vi "GPS_Air530Browser.vi"() -> ()   [LabVIEW 2024]
uses:
  <vilib>/sklein/WebView2/Webview2 Control/WebView2 Control.xctl
  Driver/CTIPicoVISA.lvlib
panel:
  out "WebView2 Control":string(xcontrol)
  out "Url":string
  out "Time Stamp":timestamp format="%<%.3X>T"
  out "Longitude":dbl format="%#_12f"
  out "Latitude":dbl format="%#_12f"
  out "$GNGGA":string
  out "error out":errorcluster
  out "NMEA Data":string="$GNGGA,100842.000,5113.89397,N,00120.47732,W,1,18,0.6,78.5,M,47.2,M,,*67\r\n$GNGLL,5113.89397,N,00120.47732,W,100842.000,A,A*56\r\n$GNGSA,A,3,01,02,03,08,10,14,17,22,27,32,,,1.0,0.6,0.8,1*30\r\n$GNGSA,A,3,12,19,20,21,22,34,35,44,,,,,1.0,0.6,0.8,4*30\r\n$GPGSV,3,1,10,01,73,289,48,02,73,0843,03,44221,35,19\r\n$PGSV,3,211,027,283,49,1722,26,302,44GPGSV,3,3,10,27,05,148,26,32,33,062,38,0*63\r\n$BDGSV,2,1,08,12,51,298,43,19,50,067,40,20,10,037,28,21,09,199,31,0*70\r\n$BDGSV,2,2,08,22,52,166,44,34,23,299,44,35,50,128,38,44,78,278,43,0*78\r\n$GNRMC,100842.000,A,5113.89397,N,00120.47732,W,0.00,0.00,130725,,,A,V*19\r\n$GNVTG,0.00,T,,M,0.00,N,0.00,K,A*23\r\n$GNZDA,100842.000,13,07,2025,00,00*47\r\n$GPTXT,01,01,01,ANTENNA OK*35\r\n$GNGGA,100843.000,5113.89397,N,00120.47732,W,1,18,0.6,78.5,M,47.2,M,,*66\r\n$GNGLL,5113.89397,N,00120.47732,W,100843.000,A,A*57\r\n$GNGSA,A,3,01,02,03,08,10,14,17,22,27,32,,,1.0,0.6,0.8,1*30\r\n$GNGSA,A,3,12,19,20,21,22,34,35,44,,,,,1.0,0.6,0.8,4*30\r\n$GPGSV,3,1,10,01,73,289,48,02,73,087,43,03,44,221,34,08,35,162,41,0*69\r\n$GPGSV,3,2,10,10,11,052,27,14,27,283,49,17,27,309,42,22,26,302,44,0*68\r\n$GPGSV,3,3,10,27,05,148,26,32,33,062,38,0*63\r\n$BDGSV,2,1,08,12,51,298,43,19,50,067,41,20,10,037,28,21,09,199,31,0*71\r\n$BDGSV,2,2,08,22,52,166,44,34,23,299,44,35,50,128,38,44,78,278,43,0*78\r\n$GNRMC,100843.000,A,5113.89397,N,00120.47732,W,0.00,0.00,130725,,,A,V*18\r\n$GNVTG,0.00,T,,M,0.00,N,0.00,K,A*23\r\n$GNZDA,100843.000,13,07,2025,00,00*46\r\n$GPTXT,01,01,01,ANTENNA OK*35\r\n$GNGGA,100844.000,5113.89397,N,00120.47732,W,1,18,0.6,78.5,M,47.2,M,,*61\r\n$GNGLL,5113.89397,N,00120.47732,W,100844.000,A,A*50\r\n$GNGSA,A,3,01,02,03,08,10,14,17,22,27,32,,,1.0,0.6,0.8,1*30\r\n$GNGSA,A,3,12,19,20,21,22,34,35,44,,,,,1.0,0.6,0.8,4*30\r\n$GPGSV,3,1,10,01,73,289,48,02,73,087,43,03,44,221,34,08,35,162,41,0*69\r\n$GPGSV,3,2,10,10,11,052,27,14,27,283,49,17,27,309,43,22,26,302,44,0*69\r\n$GPGSV,3,3,10,27,05,148,26,32,33,062,38,0*63\r\n$BDGSV,2,1,08,12,51,298,43,19,50,067,41,20,10,037,28,21,09,199,30,0*70\r\n$BDGSV,2,2,08,22,52,166,44,34,23,299,44,35,50,128,38,44,78,278,42,0*79\r\n$GNRMC,100844.000,A,5113.89397,N,00120.47732,W,0.00,0.00,130725,,,A,V*1F\r\n$GNVTG,0.00,T,,M,0.00,N,0.00,K,A*23\r\n$GNZDA,100844.000,13,07,2025,00,00*41\r\n$GPTXT,01,01,01,ANTENNA OK*35\r\n$GNGGA,100845.000,5113.89397,N,00120.47732,W,1,18,0.6,78.5,M,47.2,M,,*60\r\n$GNGLL,5113.89397,N,00120.47732,W,100845.000,A,A*51\r\n$GNGSA,A,3,01,02,03,08,10,14,17,22,27,32,,,1.0,0.6,0.8,1*30\r\n$GNGSA,A,3,12,19,20,21,22,34,35,44,,,,,1.0,0.6,0.8,4*30\r\n$GPGSV,3,1,10,01,73,289,48,02,73,087,43,03,44,221,34,08,35,162,41,0*69\r\n$GPGSV,3,2,10,10,11,052,24,14,27,283,49,17,27,309,43,22,26,302,44,0*6A\r\n$GPGSV,3,3,10,27,05,148,26,32,33,062,38,0*63\r\n$BDGSV,2,1,08,12,51,298,43,19,50,067,41,20,10,037,28,21,09,199,30,0*70\r\n$BDGSV,2,2,08,22,52,166,44,34,23,299,44,35,50,128,38,44,78,278,42,0*79\r\n$GNRMC,100845.000,A,5113.89397,N,00120.47732,W,0.00,0.00,130725,,,A,V*1E\r\n$GNVTG,0.00,T,,M,0.00,N,0.00,K,A*23\r\n$GNZDA,100845.000,13,07,202500*4PTXT01,01,01A OK*35\r$GNGGA,100846.000,5113.89397,N,00120.47732,W,1,18,0.6,78.5,M,47.2,M,,*63GLL,5113.89320.47732,W,10084A,A*52\r\nA,3,01,02,03,17,22,27,32,,,1.8,1*30\r\n$GNGSA,12,19,204,35,44,,,,,1.0,0.8,4*30V,3,1,10,01,73,28,02,73,087,43,0221,34,02,41,0*69\r\n$GPGS,10,10,124,14,27,17,309,302,44,0*6A\r\n$GP3,3,10,232,33,062,3863\r\nGSV,2,51,2989,50067,41,27,28,21,09,130,00\r\n$BDGS08,22,52,299,43,35,538,44,78,278\r\n$GNRMC,100,A,5113.89397,N,.47732,W0725,,A,V*1DG,0.00,T,,M,.00,K,A*23\r\n$GNZ.000,13,07,20*43\n$GPTXT,01,01,01,ANTENNA OK*35\r\n$GNGGA,100847.000,5113.89397,N,00120.47732,W,1,18,0.,78.2\r\n$113.10087.00,A,A3,0102,03,087,320.6,2,191,22.0,06,0.1,1001,72,73,34,3,2,17,2,05,12,598,4,27,09,1GSV,,299,35,3,0*\n$GN511397,N.00,*1C\rGNVTG,0.\r\n$GZDA,008400,001,0,ANT\r\n$GNGGA,100848.000,5113.89398,N,00120.47731W,1,,0.678.5GNGL20.4731,,100$GNG,14,7,2227,3GSA,3,1244,,0,0.V,3,,10,73,0,1621,0*3,2,50,1,27,0*60\n$GPSV,332,3,06238,098,419,57,2109,19,28,08,3,293,3578,448.0A,51,W,000,0NVTG0.0023\r\n00*4$GPT*35\r$GNGGA,1"
  in  "Len (LineTerm)":u8=4
  in  "UART Connector":enum16{"UART0", "UART1"}(ring)=enum."UART1"
  out "Identity":T1
  in  "Term Char (None)":string
  in  "Baud":u32=9600
  in  "VISA resource name in":refnum<visa-resource-name>
  in  "stop":bool
  # "https://wiki.seeedstudio.com/Grove-GPS-Air530/"
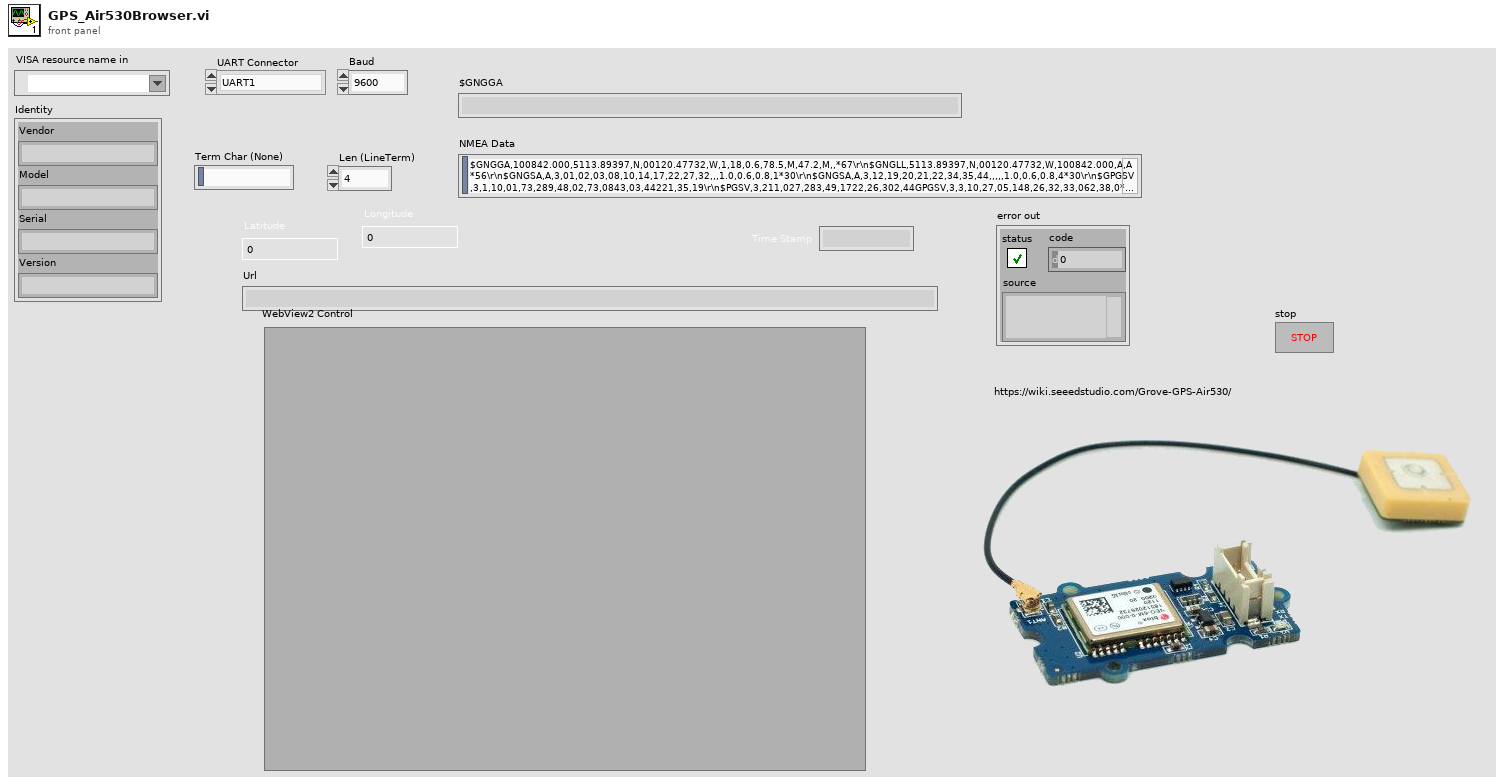
[diagram p1: front panel]
types:
  T1 = cluster{"Vendor":string, "Model":string, "Serial":string, "Version":string}
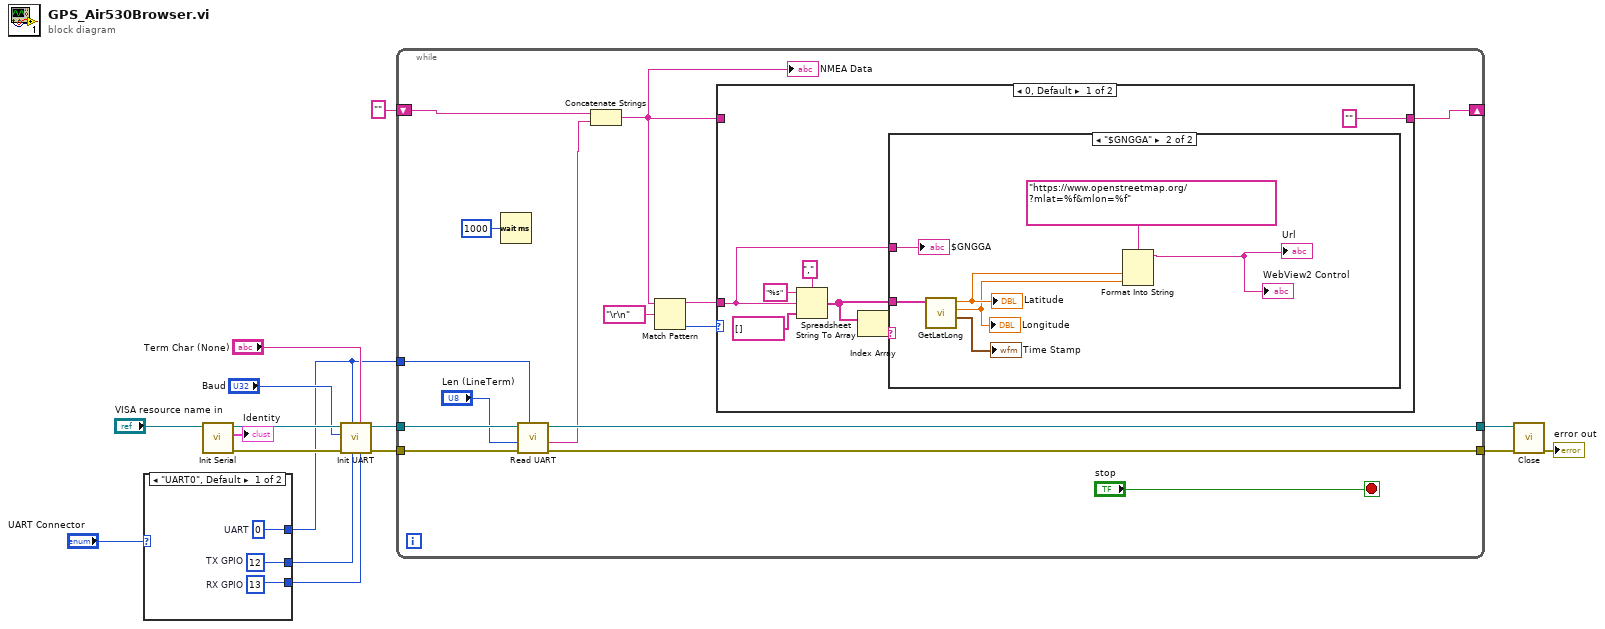
[diagram p0: block diagram]
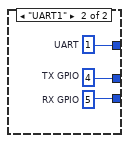
[diagram p2: hidden frame]
diagram:
  n1 = case shown="\"UART0\", Default" "UART Connector" {
    tunnel: [w19 w20] -> w9
    tunnel: [w18 w21] -> w8
    tunnel: [w17 w22] -> w7
    frame "UART0", Default {
      w18 = u8 13  # RX GPIO
      w19 = u8 12  # TX GPIO
      w17 = u8 0  # UART
    }
    frame "UART1" {
      w21 = u8 5  # RX GPIO
      w20 = u8 4  # TX GPIO
      w22 = u8 1  # UART
    }
  }
  n2 = call "Init Serial.vi"("VISA resource name in"="VISA resource name in") -> ("error out"=w14:errorcluster, "Identity"=→"Identity":T1, "VISA resource name Out"=w15:refnum<visa-resource-name>)  [unwired: 8 in]
  n3 = call "Init UART.vi"("RX GPIO"=w8, "Term Char (None)"="Term Char (None)", "TX GPIO"=w9, "UART"=w7, "error in (no error)"=w14, "Baud"="Baud", "VISA resource name in"=w15) -> ("error out"=w11:errorcluster, "VISA resource name"=w12:refnum<visa-resource-name>)  [unwired: 3 in]
  n4 = while {
    tunnel: w12 -> [w36]
    tunnel: w11 -> [w34]
    tunnel: w7 -> [w35]
    tunnel: [w31] -> w6
    tunnel: [w33] -> w5
    shift-right: [w25] -> _
    shift-left: "" -> [w32]
    stop <- "stop" stop-if-true
    n5 = Wait (ms)(milliseconds to wait=u32 1000) -> ()  [unwired: 1 out]
    n6 = call "Read UART.vi"("UART"=w35, "error in (no error)"=w34, "Len (LineTerm)"="Len (LineTerm)", "VISA resource name in"=w36) -> ("error out"=w31:errorcluster, "Data"=w29:string, "VISA resource name"=w33:refnum<visa-resource-name>)  [unwired: 5 in]
    n7 = Concatenate Strings(w32, w29) -> (w26:string)
    "NMEA Data" <- w26
    n8 = Match Pattern(string=w26, regular expression="\r\n") -> (before substring=w24:string, offset past match=w27:i32)  [unwired: 1 in, 2 out]
    n9 = case shown="0, Default" w27 {
      tunnel: w26 -> [_ w52]
      tunnel: ["" w52] -> w25
      tunnel: w24 -> [w38 _]
      frame 0, Default {
        n10 = Spreadsheet String To Array(delimiter (Tab)=",", format string="%s", spreadsheet string=w38, array type (2D Dbl)=string[] []) -> (array=w40:string[])
        n11 = Index Array(array=w40) -> (element=w39:string)  [unwired: 1 in]
        n12 = case shown="\"$GNGGA\"" w39 {
          tunnel: w40 -> [_ w51]
          tunnel: w38 -> [_ w50]
          frame "False", Default {
          }
          frame "$GNGGA" {
            n13 = call "GetLatLong.vi"("Fields"=w51) -> ("UTC Time Stamp"=→"Time Stamp":timestamp, "Longitude"=w45:dbl, "Latitude"=w46:dbl)  [unwired: 8 in]
            "Latitude" <- w46
            "Longitude" <- w45
            n14 = Format Into String(format string="https://www.openstreetmap.org/?mlat=%f&mlon=%f", w46, w45) -> (resulting string=→"Url" →"WebView2 Control":string)  [unwired: 2 in, 1 out]
            "$GNGGA" <- w50
          }
        }
      }
      frame -1 {
      }
    }
  }
  n15 = call "Close.vi"("error in (no error)"=w6, "VISA resource name in"=w5) -> ("error out"=→"error out":errorcluster)  [unwired: 9 in]
